vi "Open_PNG.vi"(4 "DRL":bool, 6 "DRR":bool, 9 "Auto L Path":path=path "C:/Program Files (x86)/CMFCD/CMFCD/data/L_Auto.PNG", 10 "Auto R Path":path=path "C:/Program Files (x86)/CMFCD/CMFCD/data/R_Auto.PNG", 11 "Aoto RL Path":path=path "C:/Program Files (x86)/CMFCD/CMFCD/data/RL_Auto.PNG") -> (3 "Knop Picture":picture)   [LabVIEW 2017]
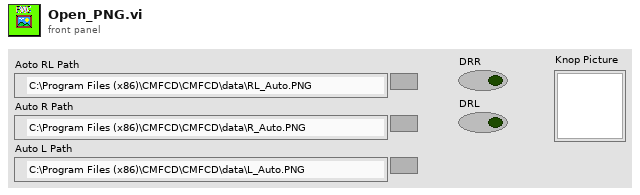
[diagram p1: front panel]
types:
  T1 = typedef "imagedata.ctl" = cluster{"image type":i32, "image depth":i32, "image":u8[], "mask":u8[], "colors":u32[], "Rectangle":cluster{"left":i16, "top":i16, "right":i16, "bottom":i16}}
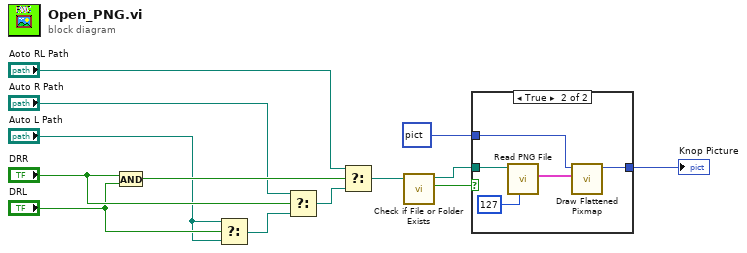
[diagram p0: block diagram]
diagram:
  n1 = And(x="DRR", y="DRL") -> (x .and. y?=w11:bool)
  n2 = Select(t="Auto L Path", s="DRL", f="Auto L Path") -> (s? t:f=w7:path)
  n3 = Select(t="Auto R Path", s="DRR", f=w7) -> (s? t:f=w9:path)
  n4 = Select(t="Aoto RL Path", s=w11, f=w9) -> (s? t:f=w4:path)
  n5 = call <vilib>:"Check if File or Folder Exists.vi"("path"=w4) -> ("file or folder exists?"=w5:bool, "dup path"=w6:path)  [unwired: 8 in, 1 out]
  n6 = case shown="True" w5 {
    tunnel: w6 -> [_ w16]
    tunnel: [w14 w18] -> w3
    tunnel: picture data[5B] ("picture") -> [w14 w17]
    frame False {
    }
    frame True {
      n7 = call <vilib>:"Read PNG File.vi"("Transparency Thresh"=u8 127, "path to PNG file"=w16) -> ("image data"=w19:T1)  [unwired: 7 in, 2 out]
      n8 = call <vilib>:"Draw Flattened Pixmap.vi"("image data"=w19, "picture"=w17) -> ("new picture"=w18:picture)  [unwired: 7 in]
    }
  }
  "Knop Picture" <- w3
